vi "Un-load.vi"(8 "error in (no error)":errorcluster, 11 "Scope(Not Paths)":T1) -> (0 "error out":errorcluster)   [LabVIEW 2020, in "ClassLoader.lvlib"]
uses:
  ClassLoader.lvlib
  Sub/Ctl/Ctl_Un-load Scope.ctl
  Sub/Ctl/Ctl_Member Map.ctl
  <vilib>/Utility/Data Type/Member VI Info.ctl
  Sub/Ctl/Ctl_PPL Details.ctl
  Sub/Cache/Cache_Members Global.vi
  Sub/Cache/Cache_Hierarchy Global.vi
  Sub/Cache/Cache_Path Global.vi
  Sub/Cache/Cache_PPL Global.vi
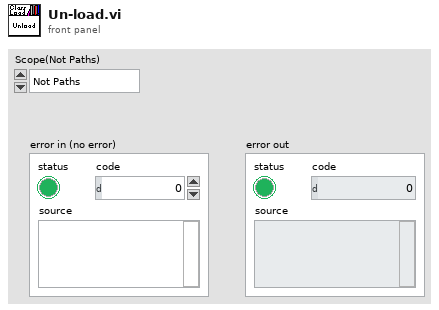
[diagram p1: front panel]
types:
  T1 = typedef "ClassLoader.lvlib/Ctl_Un-load Scope.ctl" = enum16{"Not Paths", "Not Paths nor Hierarchies", "All"}
  T2 = typedef "ClassLoader.lvlib/Ctl_Member Map.ctl" = map{string, T3}
  T3 = typedef "Member VI Info.ctl" = cluster{"qualified name":string, "path":path, "access scope":enum32{"invalid scope", "public", "private", "protected", "community"}, "is dynamic dispatch":bool}
  T4 = typedef "ClassLoader.lvlib/Ctl_PPL Details.ctl" = cluster{"Name":string, "Path":path, "Version":string}
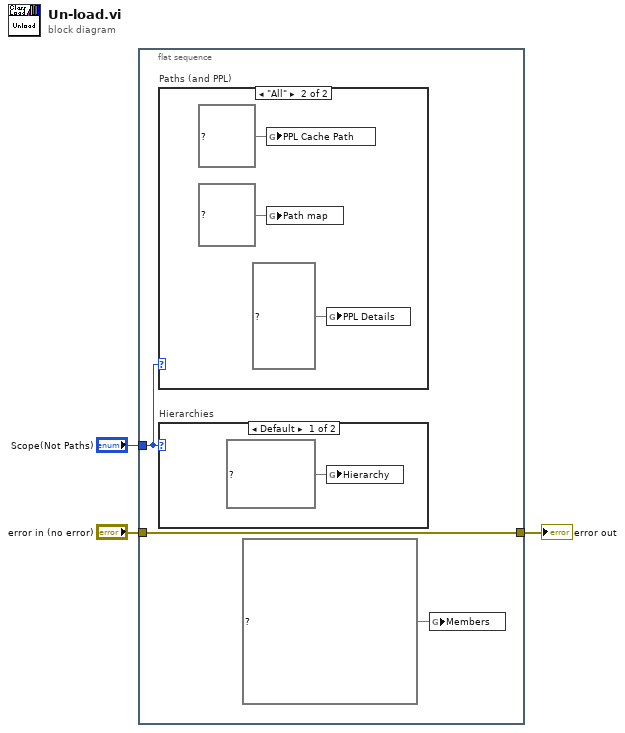
[diagram p0: block diagram]
diagram:
  n1 = flat-sequence {
    tunnel: "error in (no error)" -> [w6]
    tunnel: [w6] -> w2
    tunnel: "Scope(Not Paths)" -> [w5]
    frame #0 {
      n2 = case "Paths (and PPL)" shown="\"All\"" w5 {
        frame Default {
        }
        frame "All" {
          n3 = global write "Cache_PPL Global.vi" "PPL Cache Path"(map{string, path} {} ("PPL Cache Path")) -> ()
          n4 = global write "Cache_Path Global.vi" "Path map"(map{string, path} {} ("Path map")) -> ()
          n5 = global write "Cache_PPL Global.vi" "PPL Details"(map{string, T4} {} ("PPL Details")) -> ()
        }
      }
      n6 = case "Hierarchies" shown="Default" w5 {
        frame Default {
          n7 = global write "Cache_Hierarchy Global.vi" "Hierarchy"(map{string, string[]} {} ("Hierarchy")) -> ()
        }
        frame "Not Paths nor Hierarchies" {
        }
      }
      n8 = global write "Cache_Members Global.vi" "Members"(map{string, T2} {} ("Members")) -> ()
    }
  }
  "error out" <- w2
